vi "Write Values.vi"(8 "error in (no error)":errorcluster, 10 "Values":variant, 11 "bt_Send_Synch_WithValues in":refnum<class "bt_Send_Synch_WithValues.lvclass">) -> (0 "error out":errorcluster, 3 "bt_Send_Synch_WithValues out":refnum<class "bt_Send_Synch_WithValues.lvclass">)   [LabVIEW 2021, in "BT.lvlib" / "bt_Send_Synch_WithValues.lvclass"]
uses:
  bt_Send_Synch_WithValues.lvclass
  bt_Send_Synch_WithValues.lvclass/bt_Send_Synch_WithValues.ctl
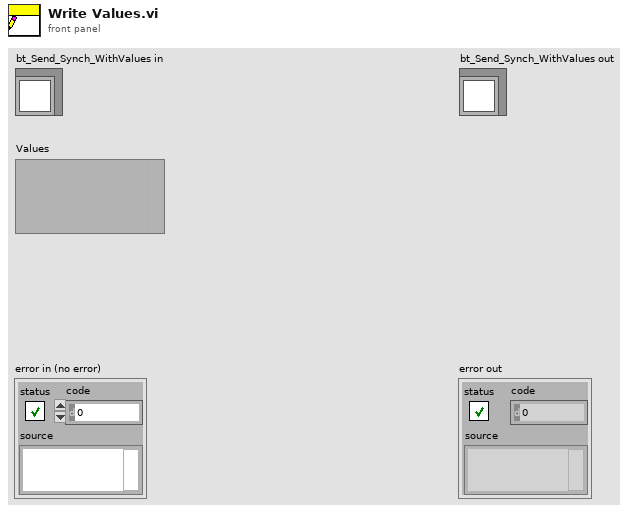
[diagram p1: front panel]
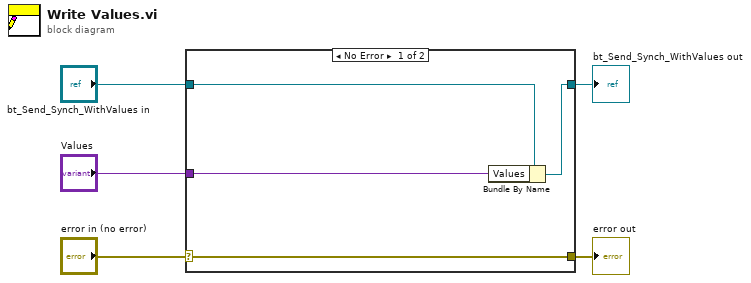
[diagram p0: block diagram]
diagram:
  n1 = case shown="No Error" "error in (no error)" {
    selector: "error in (no error)" -> [w9 w10]
    tunnel: [w9 w10] -> w4
    tunnel: [w7 w11] -> w2
    tunnel: "bt_Send_Synch_WithValues in" -> [w8 w11]
    tunnel: "Values" -> [w6 _]
    frame No Error {
      n2 = Bundle By Name(cluster=w8, "Values"=w6) -> (w7:refnum<class "bt_Send_Synch_WithValues.lvclass">)
    }
    frame Error {
    }
  }
  "error out" <- w4
  "bt_Send_Synch_WithValues out" <- w2
